vi "CoordToString.vi"(1 "coordinates":dbl[](array[numeric]) format="%.2f") -> (0 "String coordinates":string)   [LabVIEW 2013, in "File management.lvlib"]
uses:
  File management.lvlib
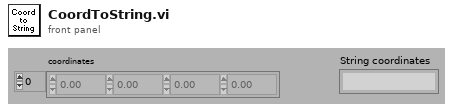
[diagram p1: front panel]
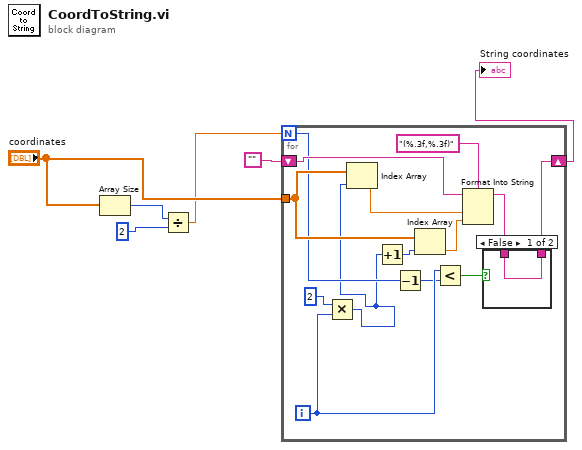
[diagram p0: block diagram]
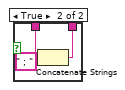
[diagram p2: hidden frame]
diagram:
  n1 = Array Size(array="coordinates") -> (size(s)=w6:i32)
  n2 = Divide(x=w6, y=2) -> (x/y=w1:dbl)
  n3 = for {
    N: w1 -> [w9]
    tunnel: "coordinates" -> [w19]
    shift-right: [w13] -> w2
    shift-left: "" -> [w17]
    i -> [w11]
    n4 = Multiply(x=2, y=w11) -> (x*y=w7:i32)
    n5 = Index Array(array=w19, index=w7) -> (element=w16:dbl)
    n6 = Increment(x=w7) -> (x+1=w12:i32)
    n7 = Decrement(x=w9) -> (x-1=w8:i32)
    n8 = Index Array(array=w19, index=w12) -> (element=w15:dbl)
    n9 = Less?(x=w11, y=w8) -> (x < y?=w10:bool)
    n10 = Format Into String(format string="(%.3f,%.3f)", initial string=w17, w16, w15) -> (resulting string=w14:string)  [unwired: 1 in, 1 out]
    n11 = case shown="False" w10 {
      tunnel: w14 -> [w21 w24]
      tunnel: [w21 w23] -> w13
      frame False {
      }
      frame True {
        n12 = Concatenate Strings(w24, " ; " ("string")) -> (w23:string)
      }
    }
  }
  "String coordinates" <- w2
